vi "GetLowerBound.vi"(8 "error in":errorcluster, 11 "RealMeasureLimit in":refnum<class "RealMeasureLimit.lvclass">) -> (0 "error out":errorcluster, 2 "LowerBound":dbl, 3 "RealMeasureLimit out":refnum<class "RealMeasureLimit.lvclass">)   [LabVIEW 2021, in "ProligentXMLGenerator.lvlib" / "RealMeasureLimit.lvclass"]
doc: "Real Measure Limit Lower Bound"
uses:
  RealMeasureLimit.lvclass
  RealMeasureLimit.lvclass/RealMeasureLimit.ctl
  Base/Decimal/Decimal.lvclass
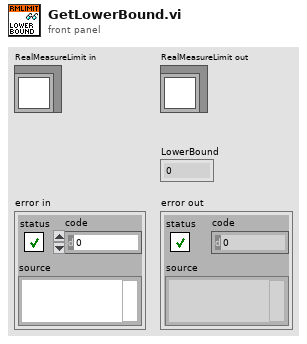
[diagram p1: front panel]
types:
  T1 = typedef "ProligentXMLGenerator.lvlib/RealMeasureLimit.lvclass/Data.ctl" = cluster{"LowerBound":refnum<class "Decimal.lvclass">, "HigherBound":refnum<class "Decimal.lvclass">}
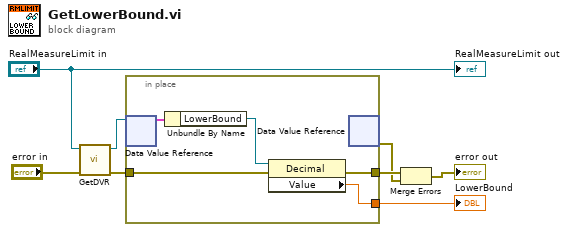
[diagram p0: block diagram]
diagram:
  n1 = call "GetDVR.vi"("error in"="error in", "RealMeasureLimit"="RealMeasureLimit in") -> ("error out"=w6:errorcluster, "DVRReference"=w5:refnum<data-value>)  [unwired: 8 in]
  n2 = in-place "In Place Element Structure" {
    in-place-border: [w9] -> w4
    in-place-border: w6 -> [w11]
    in-place-border: [w10] -> w3
    n3 = in-place-dvr #1(w5) -> (w13:T1)  [unwired: 1 out]
    n4 = Unbundle By Name(w13) -> ("LowerBound"=w12:refnum<class "Decimal.lvclass">)
    n5 = property class="Decimal"(reference=w12, error in=w11) -> (error out=w10:errorcluster, "Value"=w9:dbl)  [unwired: 1 out]
    n6 = in-place-dvr #1() -> (w1:errorcluster)  [unwired: 1 in, 1 out]
  }
  "LowerBound" <- w4
  n7 = Merge Errors(w3, w1) -> (→"error out":errorcluster)
  "RealMeasureLimit out" <- "RealMeasureLimit in"
